vi "FPGA module.vi"() -> ()   [LabVIEW 2019]
uses:
  <vilib>/Platform/TimedLoop/XDataNode/timing_clust.ctl
  <vilib>/Platform/TimedLoop/XDataNode/nitl_modes.ctl
  <vilib>/Platform/TimedLoop/XDataNode/wakeup.ctl
  <vilib>/rvi/Emulation/niFpgaGetClockAttributes.vi
  <vilib>/rvi/Emulation/niFpgaSctlEmulationGetInTimedLoop.vi
  <vilib>/rvi/Emulation/niFpgaEmulationReportErrorSimple.vi
  <vilib>/rvi/Emulation/niFpgaProcessEmulError.vi
  <vilib>/rvi/eio/common/nirviEmuTemplateMethod_errors.vi
  <vilib>/rvi/interface/RandomDataEmulation/nirviRandomDataMultiElementFPGAFIFO.vi
  <instcachedir>/0/nirviRandomDataMultiElementFPGAFIFO_1ED88BA00AC641F388A9B1FAA20E354D.lvgen/nirviRandomDataMultiElementFPGAFIFO_1ED88BA00AC641F388A9B1FAA20E354D_000.vi
  <vilib>/rvi/interface/RandomDataEmulation/niFpgaRandomDataHandleErrors.vi
  <vilib>/rvi/Emulation/niFpgaCriticalErrorInLSC.vi
  <vilib>/eio/EIONode/EIONode.xnode
  <vilib>/rvi/DataTransferAndStorage/Container/XNode/niFpgaContainer.xnode
  <vilib>/rvi/interface/RandomDataEmulation/nirviRandomDataFpgaMultiElementTemplate.vi
  <vilib>/rvi/interface/RandomDataEmulation/nirviRandomDataFpgaReadWriteTemplate.vi
  <vilib>/platform/TimedLoop/XDataNode/XDataNode.xnode
  <vilib>/Platform/TimedLoop/XDataNode/XDNodeRunTimeDep.lvlib
panel:
  out "Sum B-AI1":i32
  out "Sum B-AI0":i32
  out "ConnectorB/AI1":u16
  out "ConnectorB/AI0":u16
  out "ConnectorC/AI1":u16
  out "Sum C-AI1":i32
  out "Motor read duration":u32
  out "Generator read duration":u32
  out "Start":u32
  out "n speed":u32
  out "End":u32
  in  "Number of samples of speed":u32=1000
  out "Counter speed":u32
  in  "Number of samples":i32=100
  in  "Generator percentage":i32=1500
  in  "Motor percentage":i32=1500
  out "ConnectorA/AI3":u16
  out "Sum A-AI3":i32
  out "ConnectorC/AI0":u16
  out "Sum C-AI0":i32
  out "ConnectorA/AI2":u16
  out "Sum A-AI2":i32
  out "ConnectorA/AI1":u16
  out "Sum A-AI1":i32
  out "ConnectorA/AI0":u16
  out "n":i32
  out "Sum A-AI0":i32
  out "Bool 20kHz":bool
  in  "Counter 20kHz":i16=250
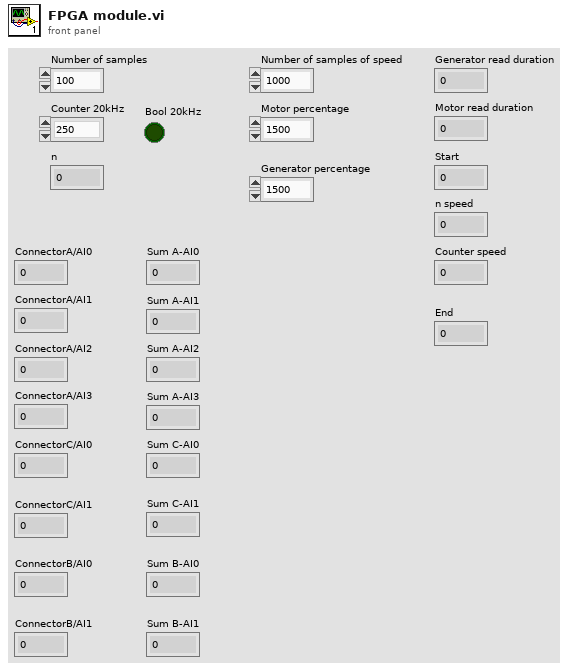
[diagram p1: front panel]
types:
  T1 = typedef "XDNodeRunTimeDep.lvlib/timing_clust.ctl" = cluster{"Expected End [f-1]":u64, "Actual End [f-1]":u64, "Finished Late? [f-1]":bool, "Expected End [i-1]":u64, "Actual End [i-1]":u64, "Finished Late? [i-1]":bool, "Expected Start [i]":u64, "Actual Start [i]":u64, "Expected Start [f]":u64, "Actual Start [f]":u64, "Source Name":string, "Structure Name":string, "Period":i64, "Deadline":i64, "Offset":i64, "Start":i64, "Priority":i32, "Timeout":i32, "Mode":T2, "Wakeup Reason":T3, "Error":errorcluster, "Source Type":string, "Secondary Source Type":string, "Global End Time":u64, "Global Start Time":u64, "Frame Duration":u64, "Iteration Duration":u64, "Assigned CPU":i32, "I/O Scan Engine Mode":u32}
  T2 = typedef "XDNodeRunTimeDep.lvlib/nitl_modes.ctl" = enum32{"No Change", "Process missed periods, maintain original phase", "Discard missed periods, maintain original phase", "Process missed periods, ignore original phase", "Discard missed periods, ignore original phase"}
  T3 = typedef "XDNodeRunTimeDep.lvlib/wakeup.ctl" = enum32{"Normal", "Aborted", "Asynchronous wakeup", "Timing source error", "Timed loop error", "Timeout"}
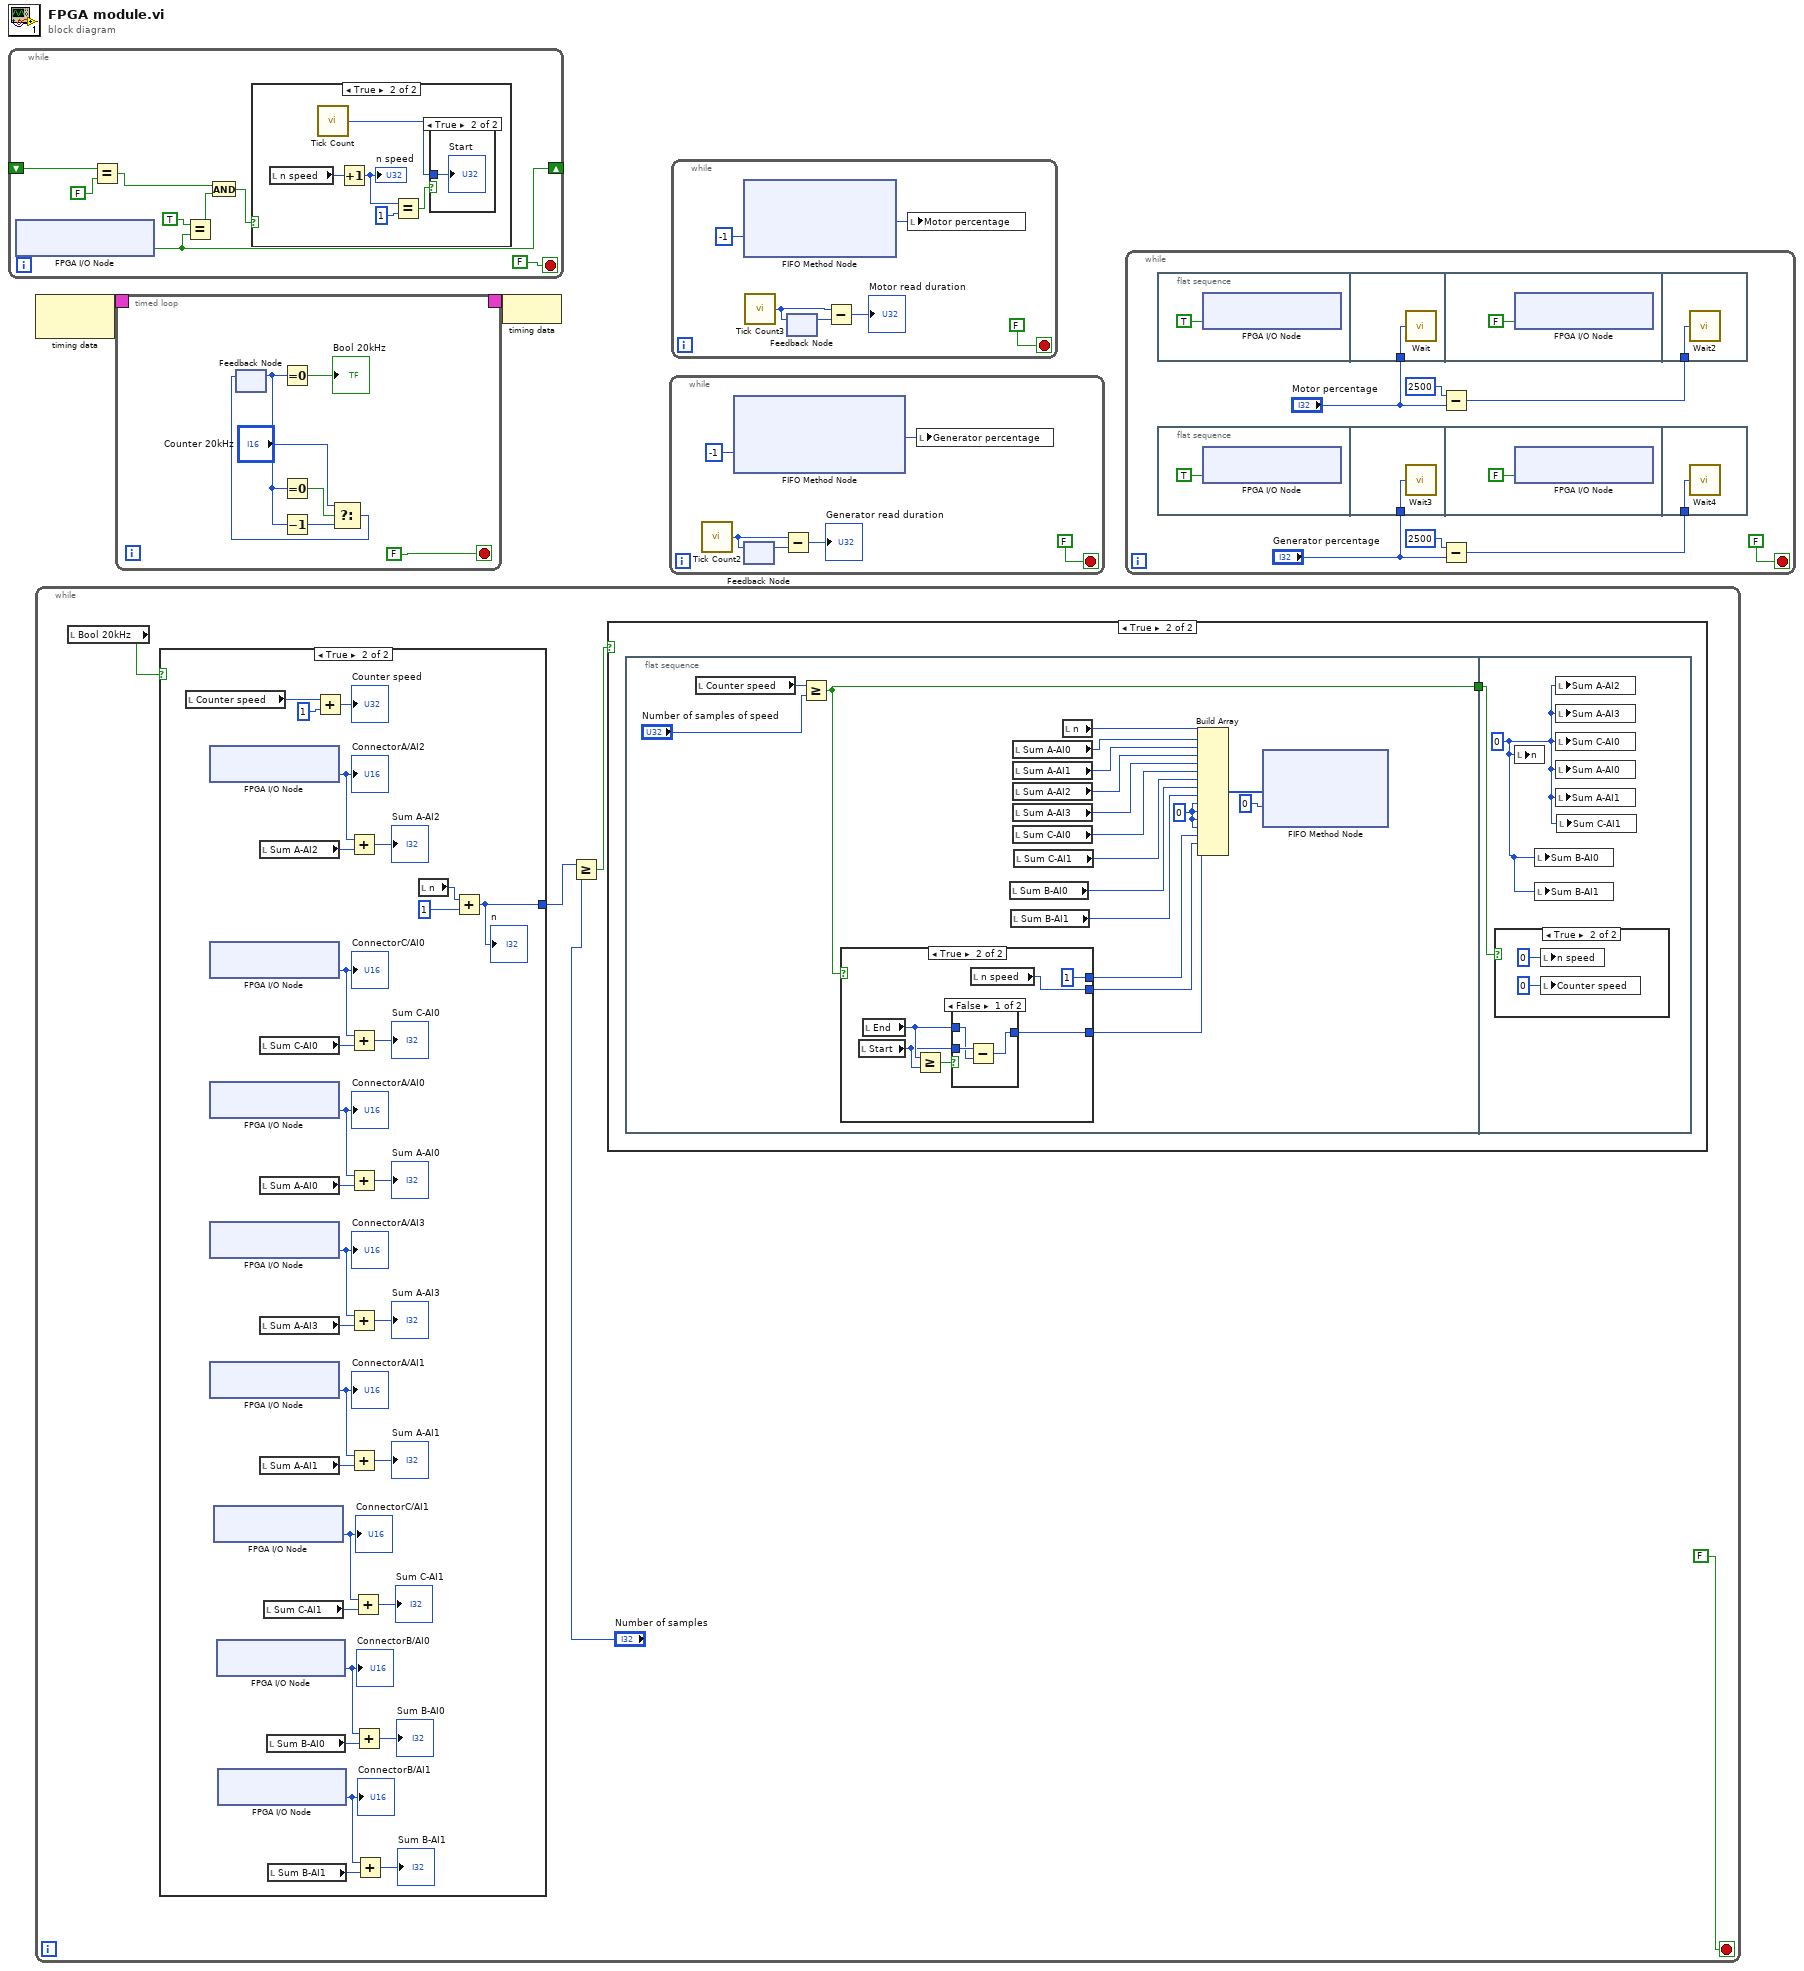
[diagram p0: block diagram]
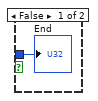
[diagram p3: hidden frame]
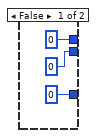
[diagram p5: hidden frame]
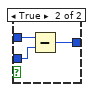
[diagram p6: hidden frame]
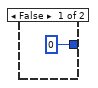
[diagram p8: hidden frame]
diagram:
  n1 = while {
    shift-right: [w6] -> _
    shift-left: _ -> [w9]
    stop <- FALSE stop-if-true
    n2 = xnode "FPGA I/O Node"() -> ("ConnectorA/DIO0"=w6:bool)  [unwired: 1 in, 1 out]
    n3 = Equal?(x=w9, y=FALSE) -> (x = y?=w5:bool)
    n4 = Equal?(x=TRUE, y=w6) -> (x = y?=w4:bool)
    n5 = And(x=w5, y=w4) -> (x .and. y?=w3:bool)
    n6 = case shown="True" w3 {
      frame False {
      }
      frame True {
        n7 = local read "n speed"() -> (w14:u32)
        n8 = call "Tick Count"() -> ("Tick Count(uSec)"=w11:u32)
        n9 = Increment(x=w14) -> (x+1=w13:u32)
        "n speed" <- w13
        n10 = Equal?(x=w13, y=u32 1) -> (x = y?=w12:bool)
        n11 = case shown="True" w12 {
          tunnel: w11 -> [w16 w17]
          frame False {
            "End" <- w16
          }
          frame True {
            "Start" <- w17
          }
        }
      }
    }
  }
  n12 = node-c288() -> (w2:T1)  [unwired: 1 in]
  n13 = while {
    stop <- FALSE stop-if-true
    n14 = local read "Bool 20kHz"() -> (w21:bool)
    n15 = case shown="True" w21 {
      tunnel: [0 w86] -> w19
      frame False {
      }
      frame True {
        n16 = local read "Counter speed"() -> (w72:u32)
        n17 = xnode "FPGA I/O Node"() -> ("ConnectorA/AI2"=w80:u16)  [unwired: 1 in, 1 out]
        "ConnectorA/AI2" <- w80
        n18 = xnode "FPGA I/O Node"() -> ("ConnectorC/AI0"=w77:i16)  [unwired: 1 in, 1 out]
        "ConnectorC/AI0" <- w77
        n19 = xnode "FPGA I/O Node"() -> ("ConnectorA/AI0"=w88:u16)  [unwired: 1 in, 1 out]
        "ConnectorA/AI0" <- w88
        n20 = xnode "FPGA I/O Node"() -> ("ConnectorA/AI3"=w74:u16)  [unwired: 1 in, 1 out]
        "ConnectorA/AI3" <- w74
        n21 = xnode "FPGA I/O Node"() -> ("ConnectorA/AI1"=w83:u16)  [unwired: 1 in, 1 out]
        "ConnectorA/AI1" <- w83
        n22 = xnode "FPGA I/O Node"() -> ("ConnectorC/AI1"=w68:i16)  [unwired: 1 in, 1 out]
        "ConnectorC/AI1" <- w68
        n23 = xnode "FPGA I/O Node"() -> ("ConnectorB/AI0"=w62:u16)  [unwired: 1 in, 1 out]
        "ConnectorB/AI0" <- w62
        n24 = xnode "FPGA I/O Node"() -> ("ConnectorB/AI1"=w67:u16)  [unwired: 1 in, 1 out]
        "ConnectorB/AI1" <- w67
        n25 = local read "Sum A-AI2"() -> (w82:i32)
        n26 = local read "Sum C-AI0"() -> (w79:i32)
        n27 = local read "Sum A-AI0"() -> (w90:i32)
        n28 = local read "Sum A-AI3"() -> (w76:i32)
        n29 = local read "Sum A-AI1"() -> (w85:i32)
        n30 = local read "Sum C-AI1"() -> (w70:i32)
        n31 = local read "Sum B-AI0"() -> (w64:i32)
        n32 = local read "Sum B-AI1"() -> (w63:i32)
        n33 = Add(x=w72, y=u32 1) -> (x+y=→"Counter speed":u32)
        n34 = Add(x=w80, y=w82) -> (x+y=→"Sum A-AI2":i32)
        n35 = Add(x=w77, y=w79) -> (x+y=→"Sum C-AI0":i32)
        n36 = Add(x=w88, y=w90) -> (x+y=→"Sum A-AI0":i32)
        n37 = Add(x=w74, y=w76) -> (x+y=→"Sum A-AI3":i32)
        n38 = Add(x=w83, y=w85) -> (x+y=→"Sum A-AI1":i32)
        n39 = Add(x=w68, y=w70) -> (x+y=→"Sum C-AI1":i32)
        n40 = Add(x=w62, y=w64) -> (x+y=→"Sum B-AI0":i32)
        n41 = Add(x=w67, y=w63) -> (x+y=→"Sum B-AI1":i32)
        n42 = local read "n"() -> (w91:i32)
        n43 = Add(x=w91, y=1) -> (x+y=w86:i32)
        "n" <- w86
      }
    }
    n44 = Greater Or Equal?(x=w19, y="Number of samples") -> (x >= y?=w20:bool)
    n45 = case shown="True" w20 {
      frame False {
      }
      frame True {
        n46 = flat-sequence {
          tunnel: [w41] -> w23
          tunnel: w23 -> [w58]
          frame #0 {
            w29 = u32 0 ("element")
            n47 = local read "Counter speed"() -> (w39:u32)
            n48 = Greater Or Equal?(x=w39, y="Number of samples of speed") -> (x >= y?=w41:bool)
            n49 = case shown="True" w41 {
              tunnel: [0 w48] -> w32
              tunnel: [0 ("n speed") w49] -> w31
              tunnel: [u32 0 ("element") u32 1 ("element")] -> w30
              frame False {
              }
              frame True {
                n50 = local read "Start"() -> (w46:u32)
                n51 = local read "End"() -> (w47:u32)
                n52 = Greater Or Equal?(x=w47, y=w46) -> (x >= y?=w45:bool)
                n53 = case shown="False" w45 {
                  tunnel: [w51 w56] -> w48
                  tunnel: w47 -> [w52 w55]
                  tunnel: w46 -> [w53 w54]
                  frame False {
                    n54 = Subtract(x=w53, y=w52) -> (x-y=w51:u32)
                  }
                  frame True {
                    n55 = Subtract(x=w55, y=w54) -> (x-y=w56:u32)
                  }
                }
                n56 = local read "n speed"() -> (w49:u32)
              }
            }
            n57 = local read "Sum B-AI0"() -> (w25:i32)
            n58 = local read "Sum B-AI1"() -> (w24:i32)
            n59 = local read "Sum A-AI0"() -> (w36:i32)
            n60 = local read "Sum A-AI1"() -> (w35:i32)
            n61 = local read "Sum A-AI2"() -> (w34:i32)
            n62 = local read "Sum A-AI3"() -> (w33:i32)
            n63 = local read "Sum C-AI0"() -> (w27:i32)
            n64 = local read "Sum C-AI1"() -> (w26:i32)
            n65 = local read "n"() -> (w37:i32)
            n66 = Build Array(w37, w36, w35, w34, w33, w27, w26, w25, w24, w29, w29, w29, w29, w30, w31, w32) -> (w28:u32[])
            n67 = xnode ("FIFO Method Node")("Element"=w28, "Timeout"=0) -> ()  [unwired: 1 in, 2 out]
          }
          frame #1 {
            w57 = 0 ("Sum A-AI0")
            n68 = case shown="True" w58 {
              frame False {
              }
              frame True {
                n69 = local write "n speed"(u32 0 ("n speed")) -> ()
                n70 = local write "Counter speed"(u32 0 ("Counter speed")) -> ()
              }
            }
            n71 = local write "n"(w57) -> ()
            n72 = local write "Sum B-AI0"(w57) -> ()
            n73 = local write "Sum B-AI1"(w57) -> ()
            n74 = local write "Sum A-AI2"(w57) -> ()
            n75 = local write "Sum A-AI3"(w57) -> ()
            n76 = local write "Sum C-AI0"(w57) -> ()
            n77 = local write "Sum A-AI0"(w57) -> ()
            n78 = local write "Sum A-AI1"(w57) -> ()
            n79 = local write "Sum C-AI1"(w57) -> ()
          }
        }
      }
    }
  }
  n80 = timed-loop {
    timing: w2 -> [_]
    timing-out: [_] -> w1
    stop <- FALSE stop-if-true
    n81 = feedback #1() -> (w95:i16)  [unwired: 1 in]
    n82 = Equal To 0?(x=w95) -> (x = 0?=→"Bool 20kHz":bool)
    n83 = Equal To 0?(x=w95) -> (x = 0?=w97:bool)
    n84 = Decrement(x=w95) -> (x-1=w96:i16)
    n85 = Select(t="Counter 20kHz", s=w97, f=w96) -> (s? t:f=w94:i16)
    n86 = feedback-in #1(w94) -> ()
  }
  n87 = node-c288(w1) -> ()
  n88 = while {
    stop <- FALSE stop-if-true
    n89 = call "Tick Count2"() -> ("Tick Count(uSec)"=w104:u32)
    n90 = xnode ("FIFO Method Node")("Timeout"=-1) -> ("Element"=w106:i32)  [unwired: 1 in, 2 out]
    n91 = feedback #2() -> (w103:u32)  [unwired: 1 in]
    n92 = feedback-in #2(w104) -> ()
    n93 = Subtract(x=w104, y=w103) -> (x-y=→"Generator read duration":u32)
    n94 = local write "Generator percentage"(w106) -> ()
  }
  n95 = while {
    stop <- FALSE stop-if-true
    n96 = xnode ("FIFO Method Node")("Timeout"=-1) -> ("Element"=w111:i32)  [unwired: 1 in, 2 out]
    n97 = call "Tick Count3"() -> ("Tick Count(uSec)"=w109:u32)
    n98 = feedback #3() -> (w108:u32)  [unwired: 1 in]
    n99 = feedback-in #3(w109) -> ()
    n100 = Subtract(x=w109, y=w108) -> (x-y=→"Motor read duration":u32)
    n101 = local write "Motor percentage"(w111) -> ()
  }
  n102 = while {
    stop <- FALSE stop-if-true
    n103 = flat-sequence {
      tunnel: "Motor percentage" -> [w125]
      tunnel: w118 -> [w127]
      frame #0 {
        n104 = xnode "FPGA I/O Node"("ConnectorA/DIO1"=TRUE ("ConnectorC/DIO3")) -> ()  [unwired: 1 in, 1 out]
      }
      frame #1 {
        n105 = call "Wait"("Count(uSec)"=w125) -> ()  [unwired: 1 out]
      }
      frame #2 {
        n106 = xnode "FPGA I/O Node"("ConnectorA/DIO1"=FALSE ("ConnectorC/DIO3")) -> ()  [unwired: 1 in, 1 out]
      }
      frame #3 {
        n107 = call "Wait2"("Count(uSec)"=w127) -> ()  [unwired: 1 out]
      }
    }
    n108 = flat-sequence {
      tunnel: "Generator percentage" -> [w121]
      tunnel: w119 -> [w123]
      frame #0 {
        n109 = xnode "FPGA I/O Node"("ConnectorA/DIO2"=TRUE ("ConnectorC/DIO3")) -> ()  [unwired: 1 in, 1 out]
      }
      frame #1 {
        n110 = call "Wait3"("Count(uSec)"=w121) -> ()  [unwired: 1 out]
      }
      frame #2 {
        n111 = xnode "FPGA I/O Node"("ConnectorA/DIO2"=FALSE ("ConnectorC/DIO3")) -> ()  [unwired: 1 in, 1 out]
      }
      frame #3 {
        n112 = call "Wait4"("Count(uSec)"=w123) -> ()  [unwired: 1 out]
      }
    }
    n113 = Subtract(x=2500, y="Motor percentage") -> (x-y=w118:i32)
    n114 = Subtract(x=2500, y="Generator percentage") -> (x-y=w119:i32)
  }
